vi "jsonInsertBool.vi"(8 "error in (no error)":errorcluster, 9 "value":bool, 10 "path":string, 11 "d in":i64) -> (0 "error out":errorcluster, 1 "replaced?":bool, 3 "d out":i64)   [LabVIEW 2015, in "JSON Document.lvclass"]
uses:
  API/JSON Document Class/JSON Document.lvclass
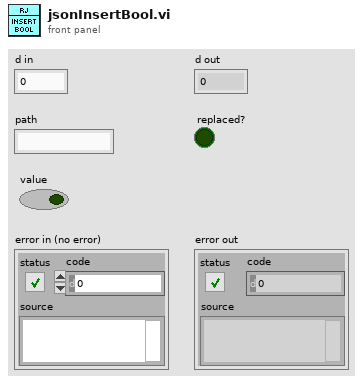
[diagram p1: front panel]
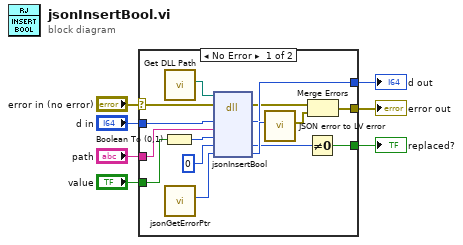
[diagram p0: block diagram]
diagram:
  n1 = case shown="No Error" "error in (no error)" {
    selector: "error in (no error)" -> [w14 w24]
    tunnel: [w11 w24] -> w7
    tunnel: "value" -> [w18 _]
    tunnel: "d in" -> [w17 w23]
    tunnel: "path" -> [w16 _]
    tunnel: [w15 w23] -> w2
    tunnel: [w8 _] -> w1
    frame No Error {
      n2 = Boolean To (0,1)(Boolean=w18) -> (0, 1=w19:i16)
      n3 = call "Get DLL Path.vi"() -> ("Path"=w22:path)  [unwired: 11 in]
      n4 = call "jsonGetErrorPtr.vi"() -> ("return type"=w20:i64)  [unwired: 10 in, 1 out]
      n5 = dll-call lib="C:/Users/tblair/Documents/Git Projects/rapidjson-for-LabVIEW/lvrjs/Debug/lvrjs.dll" fn="jsonInsertBool"(path in=w22, error in=w14, "d"=w17, "path"=w16, "value"=w19, "replaced"=0, "jsonError"=w20) -> (error out=w13:errorcluster, "d"=w15:i64, "replaced"=w9:i32, "jsonError"=w21:i64)  [unwired: 4 in, 1 out]
      n6 = call "JSON error to LV error.vi"("jsonError"=w21) -> ("error out"=w12:errorcluster)  [unwired: 10 in]
      n7 = Not Equal To 0?(x=w9) -> (x != 0?=w8:bool)
      n8 = Merge Errors(w13, w12) -> (w11:errorcluster)
    }
    frame Error {
    }
  }
  "error out" <- w7
  "d out" <- w2
  "replaced?" <- w1
